vi "Test Split.vi"() -> ()   [LabVIEW 2024, in "Spectrum Recorder too.lvclass"]
uses:
  Spectrum Recorder too.lvclass
  NHMFL_Core/Libraries/Red Pitaya/RP Core/RP Instrument/RP Instrument.lvclass
  NHMFL_Core/Libraries/Red Pitaya/RP Core/RP Instrument/RP Instrument.lvclass/RP Instrument.ctl
  NHMFL_Core/Libraries/Red Pitaya/RP Core/RP Instrument/Write bytes per RX sample.vi
  NHMFL_Core/Libraries/Red Pitaya/RP Core/RP Instrument/Write Server address.vi
panel:
  out "In":i32[](array[numeric])
  in  "Reset TX":bool
  in  "Scale":i32=10
  in  "Firmware":enum16{"Split test", "Desimation"}(ring)
  in  "Red Pitaya address":string="192.168.1.120"
  in  "milliseconds to wait":u32=1000
  out "Waveform Graph":i32[][](graph)
  in  "N point in":i32=1024 format="0x%x (%d)"
  out "X counter":i32=32
  out "y counter":u32=3002 format="0x%x (%d)"
  out "Y":i32[](array[numeric])
  out "X":i32[](array[numeric])
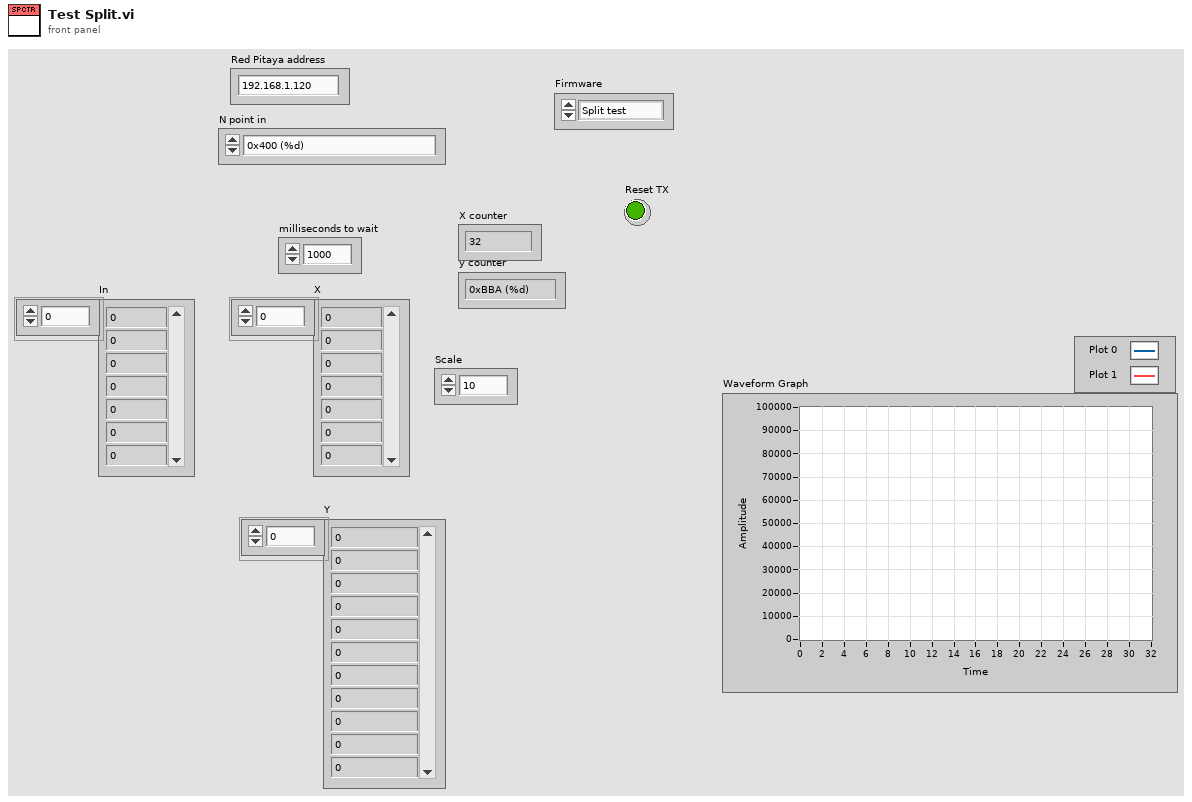
[diagram p1: front panel]
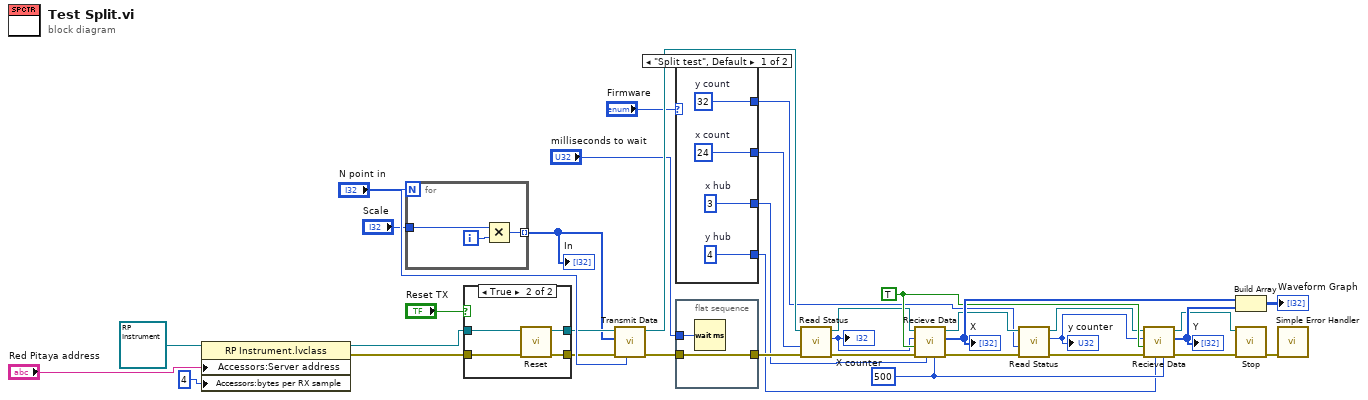
[diagram p0: block diagram]
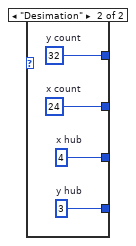
[diagram p3: hidden frame]
diagram:
  w14 = 500 ("timeout ms (25000)")
  w32 = TRUE ("Force read")
  n1 = property class="RP Instrument.lvclass"(reference=refnum<class "RP Instrument.lvclass"> refnum ("RP Instrument.lvclass"), "Accessors:Server address"="Red Pitaya address", "Accessors:bytes per RX sample"=u32 4 ("bytes per RX sample")) -> (reference out=w6:refnum<class "RP Instrument.lvclass">, error out=w4:errorcluster)  [unwired: 1 in]
  n2 = for {
    N: "N point in" -> [_]
    tunnel: [w38] -> w1 mode=indexing
    tunnel: "Scale" -> [w37]
    i -> [w39]
    n3 = Multiply(x=w37, y=w39) -> (x*y=w38:i32)
  }
  "In" <- w1
  n4 = case shown="True" "Reset TX" {
    tunnel: w6 -> [w40 w45]
    tunnel: [w40 w44] -> w5
    tunnel: w4 -> [w41 w43]
    tunnel: [w41 w42] -> w3
    frame False {
    }
    frame True {
      n5 = call-dynamic "Reset.vi"("error in (no error)"=w43, "RP Instrument in"=w45) -> ("error out"=w42:errorcluster, "RP Instrument out"=w44:refnum<class "RP Instrument.lvclass">)  [unwired: 8 in]
    }
  }
  n6 = call-dynamic "Transmit Data.vi"("Buffer size"="N point in", "error in (no error)"=w3, "Data"=w1, "RP Instrument in"=w5) -> ("error out"=w18:errorcluster, "RP Instrument out"=w30:refnum<class "RP Instrument.lvclass">)  [unwired: 6 in]
  n7 = case shown="\"Split test\", Default" "Firmware" {
    tunnel: [w49 w53] -> w11
    tunnel: [w48 w52] -> w10
    tunnel: [w47 w51] -> w9
    tunnel: [w46 w50] -> w8
    frame "Split test", Default {
      w46 = u64 32  # y count
      w47 = u64 24  # x count
      w48 = u64 4  # y hub
      w49 = u64 3  # x hub
    }
    frame "Desimation" {
      w50 = u64 32  # y count
      w51 = u64 24  # x count
      w52 = u64 3  # y hub
      w53 = u64 4  # x hub
    }
  }
  n8 = flat-sequence {
    tunnel: w18 -> [w55]
    tunnel: [w55] -> w17
    tunnel: "milliseconds to wait" -> [w54]
    frame #0 {
      n9 = Wait (ms)(milliseconds to wait=w54) -> ()  [unwired: 1 out]
    }
  }
  n10 = call-dynamic "Read Status.vi"("error in (no error)"=w17, "Status offset"=w9, "RP Instrument in"=w30) -> ("error out"=w27:errorcluster, "Status response"=w29:u32, "RP Instrument out"=w28:refnum<class "RP Instrument.lvclass">)  [unwired: 6 in]
  "X counter" <- w29
  n11 = call-dynamic "Recieve Data.vi"("timeout ms (25000)"=w14, "hub port"=w11, "error in (no error)"=w27, "Force read"=w32, "Points to read"=w29, "RP Instrument in"=w28) -> ("error out"=w26:errorcluster, "Data out"=w35:i32[], "RP Instrument out"=w24:refnum<class "RP Instrument.lvclass">)  [unwired: 3 in]
  "X" <- w35
  n12 = call-dynamic "Read Status.vi"("error in (no error)"=w26, "Status offset"=w8, "RP Instrument in"=w24) -> ("error out"=w25:errorcluster, "Status response"=w22:u32, "RP Instrument out"=w23:refnum<class "RP Instrument.lvclass">)  [unwired: 6 in]
  "y counter" <- w22
  n13 = call-dynamic "Recieve Data.vi"("timeout ms (25000)"=w14, "hub port"=w10, "error in (no error)"=w25, "Force read"=w32, "Points to read"=w22, "RP Instrument in"=w23) -> ("error out"=w20:errorcluster, "Data out"=w34:i32[], "RP Instrument out"=w21:refnum<class "RP Instrument.lvclass">)  [unwired: 3 in]
  "Y" <- w34
  n14 = Build Array(w35, w34) -> (→"Waveform Graph":i32[][])
  n15 = call-dynamic "Stop.vi"("error in (no error)"=w20, "RP Instrument in"=w21) -> ("error out"=w19:errorcluster)  [unwired: 8 in, 1 out]
  n16 = call <vilib>:"Simple Error Handler.vi"("error in (no error)"=w19) -> ()  [unwired: 4 in, 5 out]
